vi "Cleanup.vi"(8 "error in (no error)":errorcluster, 11 "VoiceMeeterRemote in":refnum<class "VoiceMeeterRemote.lvclass">) -> (0 "error out":errorcluster)   [LabVIEW 2022 SP3, in "VoiceMeeterRemote.lvlib" / "VoiceMeeterRemote.lvclass"]
uses:
  VoiceMeeterRemote.lvclass
  VoiceMeeterRemote.lvclass/VoiceMeeterRemote.ctl
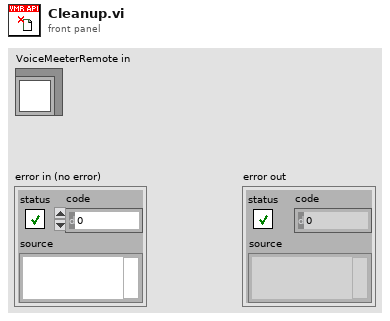
[diagram p1: front panel]
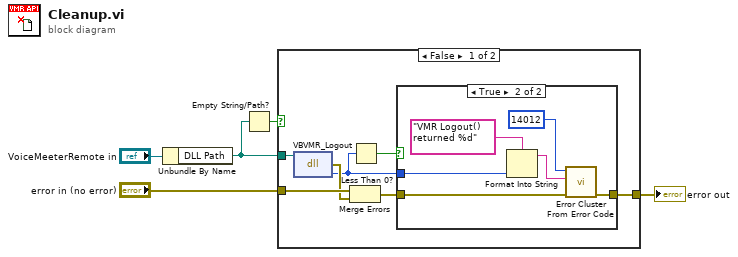
[diagram p0: block diagram]
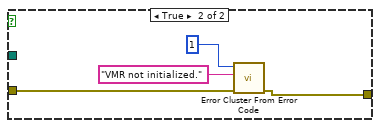
[diagram p3: hidden frame]
diagram:
  n1 = Unbundle By Name("VoiceMeeterRemote in") -> ("DLL Path"=w2:path)
  n2 = Empty String/Path?(string/path=w2) -> (empty?=w1:bool)
  n3 = case shown="False" w1 {
    tunnel: "error in (no error)" -> [w12 w23]
    tunnel: [w7 w22] -> w4
    tunnel: w2 -> [w6 _]
    frame False {
      n4 = dll-call lib="C:/Program Files/National Instruments/LabVIEW 2022/user.lib/VoicemeeterRemote64/VoicemeeterRemote64.*" fn="VBVMR_Logout"(path in=w6) -> (error out=w11:errorcluster, "return type"=w10:i32)  [unwired: 2 in, 1 out]
      n5 = Merge Errors(w12, w11) -> (w9:errorcluster)
      n6 = Less Than 0?(x=w10) -> (x < 0?=w8:bool)
      n7 = case shown="True" w8 {
        tunnel: w10 -> [_ w17]
        tunnel: w9 -> [w13 w19]
        tunnel: [w13 w14] -> w7
        frame False {
        }
        frame True {
          n8 = Format Into String(format string="VMR Logout() returned %d", w17) -> (resulting string=w15:string)  [unwired: 2 in, 1 out]
          n9 = call <vilib>:"Error Cluster From Error Code.vi"("error in (no error)"=w19, "error message (\"\")"=w15, "error code (0)"=14012) -> ("error out"=w14:errorcluster)  [unwired: 6 in]
        }
      }
    }
    frame True {
      n10 = call <vilib>:"Error Cluster From Error Code.vi"("error in (no error)"=w23, "error message (\"\")"="VMR not initialized." ("error message (\"\")"), "error code (0)"=1) -> ("error out"=w22:errorcluster)  [unwired: 6 in]
    }
  }
  "error out" <- w4
